vi "MenuItem_Create.vi"(6 "Isveg":bool, 7 "Price":dbl, 8 "Error In":errorcluster, 9 "Description":string, 10 "Name":string, 11 "reference in":refnum<class "MenuItem.lvclass">) -> (0 "Error Out":errorcluster, 3 "reference out":refnum<class "MenuItem.lvclass">)   [LabVIEW 2020, in "MenuItem.lvclass"]
uses:
  MenuItem.lvclass
  C:/Projects/OpenGDS_DesignPatterns/Composition1/MenuComponent_class/MenuComponent.lvclass
  MenuComponent_class/MenuComponent.lvclass
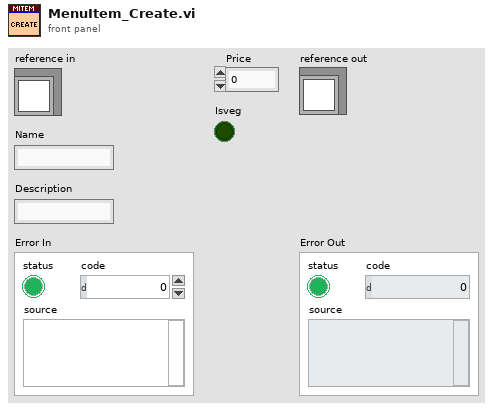
[diagram p1: front panel]
types:
  T1 = typedef "MenuItem.lvclass/ObjectAttributes.ctl" = cluster{"Name":string, "Description":string, "Price":dbl, "Vegetarian":bool}
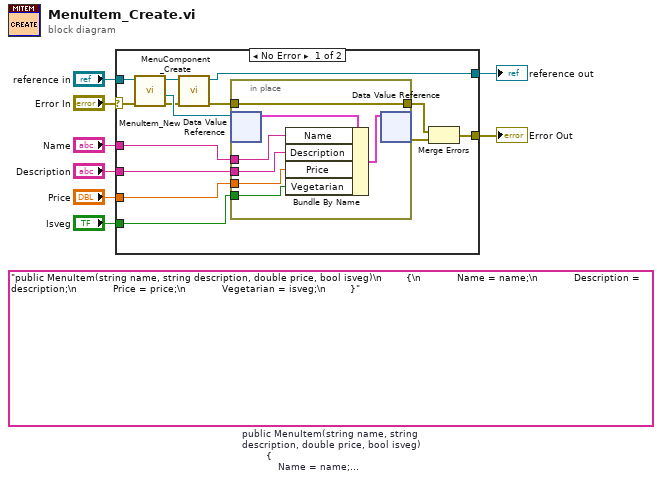
[diagram p0: block diagram]
diagram:
  (unwired) "public MenuItem(string name, string description, double price, bool isveg)\n        {\n            Name = name;\n            Description = description;\n            Price = price;\n            Vegetarian = isveg;\n        }"  # public MenuItem(string name, string description, double price, bool isveg)         {             Name = name;             Description = description;             Price = price;             Vegetarian = isveg;         }
  n1 = case shown="No Error" "Error In" {
    selector: "Error In" -> [w18 w31]
    tunnel: [w16 w31] -> w7
    tunnel: "reference in" -> [w20 w30]
    tunnel: [w15 w30] -> w5
    tunnel: "Price" -> [w12 _]
    tunnel: "Name" -> [w11 _]
    tunnel: "Description" -> [w10 _]
    tunnel: "Isveg" -> [w9 _]
    frame No Error {
      n2 = call "MenuItem_New.vi"("error in (no error)"=w18, "reference in"=w20) -> ("error out"=w19:errorcluster, "DVRRefOut"=w22:refnum<data-value>, "reference out"=w21:refnum<class "MenuItem.lvclass">)  [unwired: 6 in, 1 out]
      n3 = call "MenuComponent_Create.vi"("Error In"=w19, "reference in"=w21) -> ("Error Out"=w14:errorcluster, "reference out"=w15:refnum<class "MenuItem.lvclass">)  [unwired: 8 in]
      n4 = in-place {
        in-place-border: w14 -> [w27]
        in-place-border: [w27] -> w13
        in-place-border: w12 -> [w26]
        in-place-border: w11 -> [w25]
        in-place-border: w10 -> [w24]
        in-place-border: w9 -> [w23]
        n5 = in-place-dvr #1(w22) -> (w28:T1)  [unwired: 1 out]
        n6 = Bundle By Name(cluster=w28, "Name"=w25, "Description"=w24, "Price"=w26, "Vegetarian"=w23) -> (w29:T1)
        n7 = in-place-dvr #1(w29) -> (w17:errorcluster)  [unwired: 1 out]
      }
      n8 = Merge Errors(w13, w17) -> (w16:errorcluster)
    }
    frame Error {
    }
  }
  "Error Out" <- w7
  "reference out" <- w5
